vi "New FPGATarget2.vi"(8 "bitfile contents":string, 9 "target location":string) -> (3 "session":u32)   [LabVIEW 2020, in "NI_TargetHelper.lvlib"]
uses:
  <vilib>/TargetSupport/NI_TargetHelper/NI_TargetHelper.lvlib
  <vilib>/rvi/ClientSDK/nirviWhatTheDeviceIsDoing.ctl
  NiFpgaLv.dll
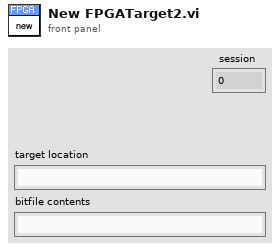
[diagram p1: front panel]
types:
  T1 = typedef "nirviWhatTheDeviceIsDoing.ctl" = enum32{"C Interface", "RIO Scan Interface", "FPGA interface", "Interactive Mode", "Emulation Mode"}
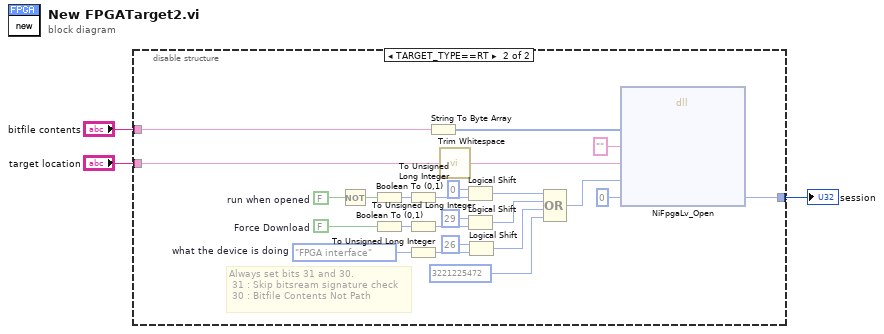
[diagram p0: block diagram]
diagram:
  n1 = disable-structure shown="TARGET_TYPE==RT" {
    disable-tunnel: "bitfile contents" -> [_ w6]
    disable-tunnel: "target location" -> [_ w5]
    disable-tunnel: [_ w4] -> w1
    frame condition #0 (active) {
    }
    frame condition #1 {
      w26 = nirviWhatTheDeviceIsDoing."FPGA interface"  # what the device is doing
      w13 = FALSE  # Force Download
      w14 = FALSE  # run when opened
      # "Always set bits 31 and 30.\n 31 : Skip bitsream signature check\n 30 : Bitfile Contents Not Path"
      n2 = Not(x=w14) -> (.not. x?=w15:bool)
      n3 = Boolean To (0,1)(Boolean=w15) -> (0, 1=w8:i16)
      n4 = Boolean To (0,1)(Boolean=w13) -> (0, 1=w18:i16)
      n5 = To Unsigned Long Integer(number=w8) -> (unsigned 32bit integer=w7:u32)
      n6 = To Unsigned Long Integer(number=w18) -> (unsigned 32bit integer=w20:u32)
      n7 = To Unsigned Long Integer(number=w26) -> (unsigned 32bit integer=w22:u32)
      n8 = String To Byte Array(string=w6) -> (unsigned byte array=w12:u8[])
      n9 = call <vilib>:"Trim Whitespace.vi"("string"=w5) -> ("trimmed string"=w11:string)  [unwired: 1 in]
      n10 = Logical Shift(y=u32 0 ("x"), x=w7) -> (x << y=w9:u32)
      n11 = Logical Shift(y=u32 29 ("x"), x=w20) -> (x << y=w17:u32)
      n12 = Logical Shift(y=u32 26 ("x"), x=w22) -> (x << y=w25:u32)
      n13 = Compound Arithmetic op=OR(w9, w17, w25, u32 3221225472 ("x")) -> (w24:u32)
      n14 = dll-call lib="NiFpgaLv.*" fn="NiFpgaLv_Open" label="niLvFpgaOpen"("bitfileInfo"=w12, "apiSignature"="", "resource"=w11, "attribute"=w24, "session"=u32 0 ("session in")) -> ("session"=w4:u32)  [unwired: 5 in, 5 out]
    }
  }
  "session" <- w1
